vi "BubbleSort.vi"(11 "LinkedList in":T1) -> (3 "LinkedList out":T1)   [LabVIEW 2010]
uses:
  LinkedList.ctl
  Node.ctl
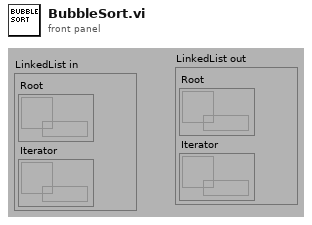
[diagram p1: front panel]
types:
  T1 = typedef "LinkedList.ctl" = cluster{"Root":refnum<data-value>, "Iterator":refnum<data-value>}
  T2 = typedef "Node.ctl" = cluster{"Name":string, "Next":variant, "Previous":variant}
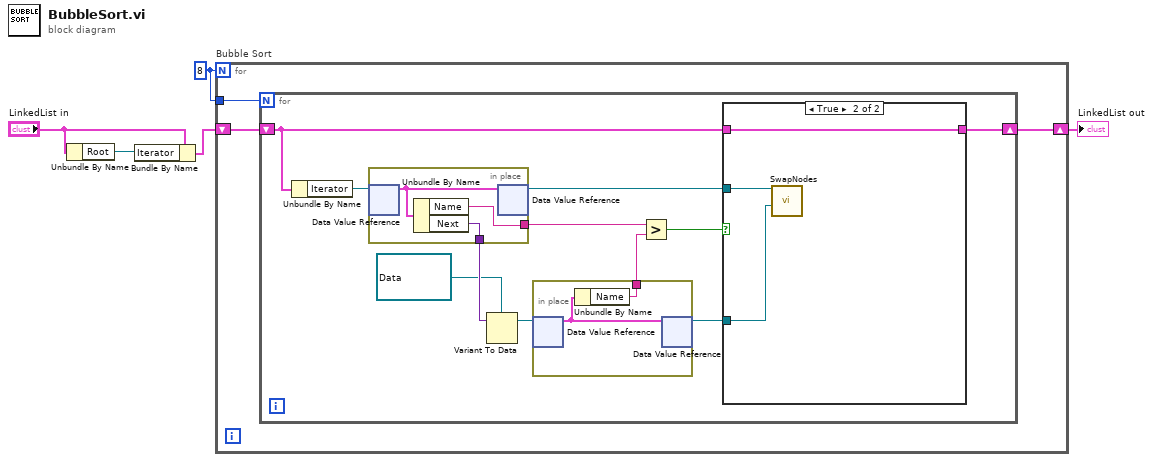
[diagram p0: block diagram]
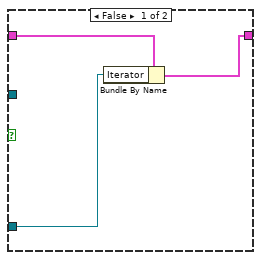
[diagram p2: hidden frame]
diagram:
  w5 = 8
  n1 = Unbundle By Name("LinkedList in") -> ("Root"=w2:refnum<data-value>)
  n2 = Bundle By Name(cluster="LinkedList in", "Iterator"=w2) -> (w4:T1)
  n3 = for "Bubble Sort" {
    N: w5 -> [_]
    shift-right: [w7] -> w1
    shift-left: w4 -> [w8]
    tunnel: w5 -> [w6]
    n4 = for {
      N: w6 -> [_]
      shift-right: [w9] -> w7
      shift-left: w8 -> [w10]
      n5 = Unbundle By Name(w10) -> ("Iterator"=w19:refnum<data-value>)
      n6 = in-place {
        in-place-border: [w30] -> w18
        in-place-border: [w28] -> w15
        n7 = in-place-dvr #1(w19) -> (w29:T2)  [unwired: 1 out]
        n8 = Unbundle By Name(w29) -> ("Name"=w28:string, "Next"=w30:variant)
        n9 = in-place-dvr #1(w29) -> (w12:refnum<data-value>)  [unwired: 1 out]
      }
      n10 = Variant To Data(Variant=w18, type=refnum<data-value> refnum ("data value reference")) -> (data=w16:refnum<data-value>)  [unwired: 1 in, 1 out]
      n11 = in-place {
        in-place-border: [w27] -> w14
        n12 = in-place-dvr #2(w16) -> (w26:T2)  [unwired: 1 out]
        n13 = Unbundle By Name(w26) -> ("Name"=w27:string)
        n14 = in-place-dvr #2(w26) -> (w11:refnum<data-value>)  [unwired: 1 out]
      }
      n15 = Greater?(x=w15, y=w14) -> (0:w13:bool)
      n16 = case shown="True" w13 {
        tunnel: w12 -> [_ w25]
        tunnel: w11 -> [w21 w24]
        tunnel: w10 -> [w22 w23]
        tunnel: [w20 w23] -> w9
        frame False {
          n17 = Bundle By Name(cluster=w22, "Iterator"=w21) -> (w20:T1)
        }
        frame True {
          n18 = call "SwapNodes.vi"("Node2"=w24, "Node1"=w25) -> ()  [unwired: 10 in]
        }
      }
    }
  }
  "LinkedList out" <- w1
